vi "Subscribe to Panel Resized.vi"(8 "error in":errorcluster, 9 "Message":refnum<class "Message.lvclass">, 10 "Enqueuer":refnum<class "Message Enqueuer.lvclass">, 11 "Flex  Dialog (Actor) in":refnum<class "Flex Dialog (Actor).lvclass">) -> (0 "error out":errorcluster, 3 "Flex  Dialog (Actor) out":refnum<class "Flex Dialog (Actor).lvclass">)   [LabVIEW 2016, in "Flex UI Dialog (Actor).lvlib" / "Flex Dialog (Actor).lvclass"]
uses:
  Flex Dialog (Actor).lvclass
  <vilib>/ActorFramework/Message/Message.lvclass
  <vilib>/ActorFramework/Message Enqueuer/Message Enqueuer.lvclass
  <vilib>/East West Architects/MVC Subscription/Subscription/MVC Subscription.lvclass
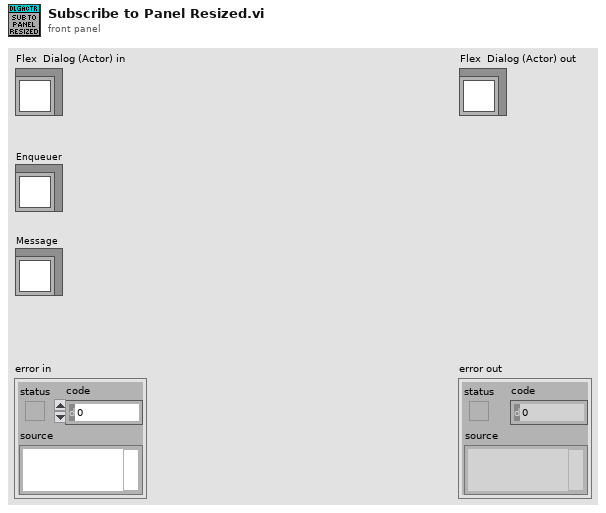
[diagram p1: front panel]
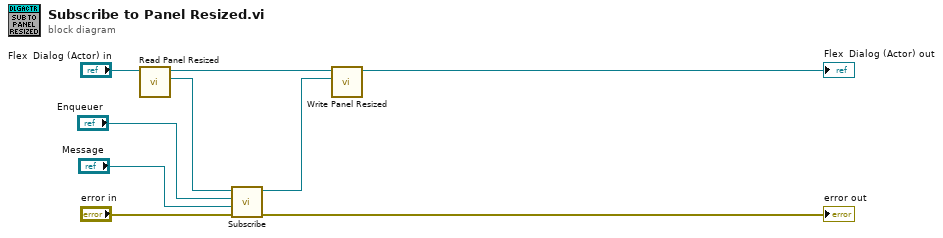
[diagram p0: block diagram]
diagram:
  n1 = call-dynamic "Read Panel Resized.vi"("Flex  Dialog (Actor) in"="Flex  Dialog (Actor) in") -> ("Panel Resized"=w4:refnum<class "MVC Subscription.lvclass">, "Flex  Dialog (Actor) out"=w7:refnum<class "Flex Dialog (Actor).lvclass">)  [unwired: 9 in]
  n2 = call <vilib>:"Subscribe.vi"("error in"="error in", "Message"="Message", "Enqueuer"="Enqueuer", "MVC Subscription in"=w4) -> ("error out"=→"error out":errorcluster, "MVC Subscription out"=w3:refnum<class "MVC Subscription.lvclass">)  [unwired: 6 in]
  n3 = call-dynamic "Write Panel Resized.vi"("Panel Resized"=w3, "Flex  Dialog (Actor) in"=w7) -> ("Flex  Dialog (Actor) out"=→"Flex  Dialog (Actor) out":refnum<class "Flex Dialog (Actor).lvclass">)  [unwired: 9 in]
